vi "SR_400_count_with_trigger.vi"() -> ()   [LabVIEW 2015]
uses:
  Libraries/SR400/SR400.lvlib
  Downloads/SRS SR400/SRS SR400.lvlib
panel:
  in  "SR_400_GPIB_ADDR":refnum<visa-resource-name>="GPIB0::18::INSTR"
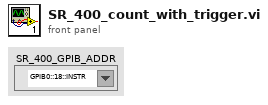
[diagram p1: front panel]
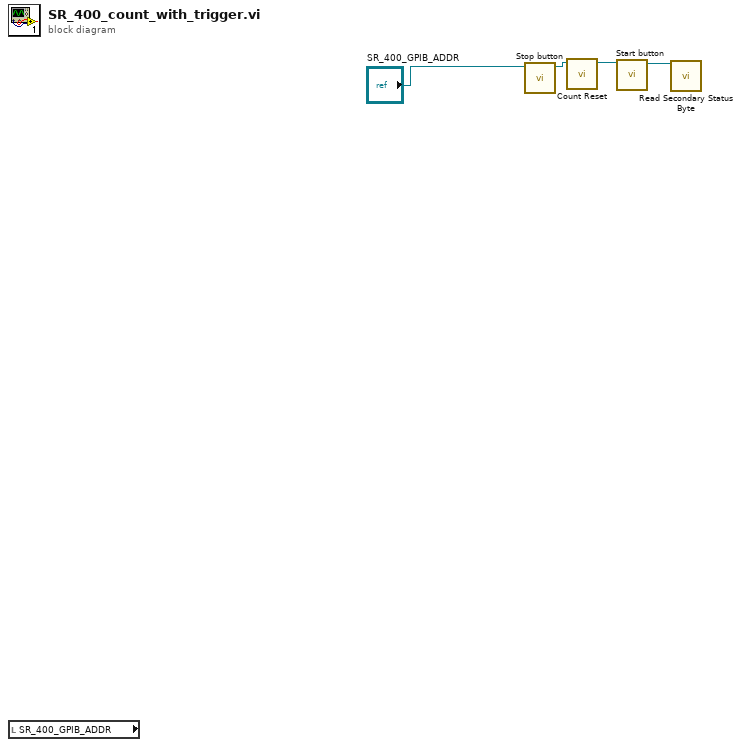
[diagram p0: block diagram]
diagram:
  n1 = local read "SR_400_GPIB_ADDR"() -> (w2:refnum<visa-resource-name>)
  n2 = call "Stop button.vi"("VISA resource name"="SR_400_GPIB_ADDR") -> ("VISA resource name out"=w5:refnum<visa-resource-name>)  [unwired: 9 in, 1 out]
  n3 = call "Count Reset.vi"("VISA resource name"=w5) -> ("VISA resource name out"=w4:refnum<visa-resource-name>)  [unwired: 9 in, 1 out]
  n4 = call "Start button.vi"("VISA resource name"=w4) -> ("VISA resource name out"=w3:refnum<visa-resource-name>)  [unwired: 9 in, 1 out]
  n5 = call "Read Secondary Status Byte.vi"("VISA resource name"=w3) -> ()  [unwired: 7 in, 4 out]
